vi "DeltaYonDeltaX.vi"() -> (0 "New Values In":string[][](array[string])=[["Test data5"]], 1 "New Chs In":string[](array[string])=["30-10-03:New:Channel new5"])   [LabVIEW 2022 SP3]
uses:
  Results_plotter_Global.vi
  Data plotting/subVIs/Plot_Values_Global.vi
panel:
  # "Similar to Calculate_Gradient.vi, but also returns sign. However does not cope with multiple ordinates."
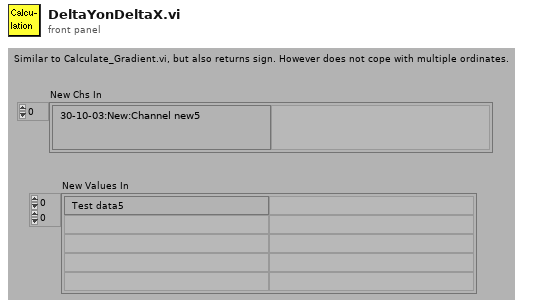
[diagram p1: front panel]
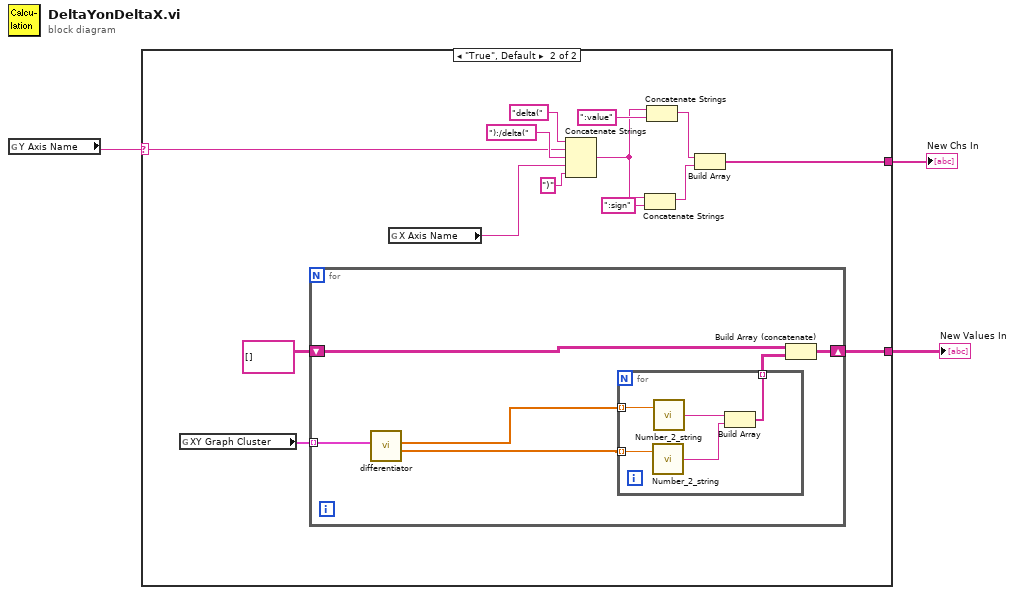
[diagram p0: block diagram]
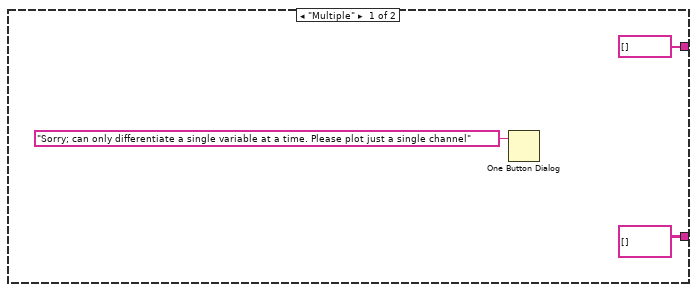
[diagram p2: hidden frame]
diagram:
  n1 = global read "Results_plotter_Global.vi" "Y Axis Name"() -> (w1:string)
  n2 = case shown="\"True\", Default" w1 {
    selector: w1 -> [_ w7]
    tunnel: [string[][] [] w19] -> w3
    tunnel: [string[] [] w11] -> w2
    frame "Multiple" {
      n3 = One Button Dialog(message="Sorry; can only differentiate a single variable at a time. Please plot just a single channel") -> ()  [unwired: 1 in, 1 out]
    }
    frame "True", Default {
      n4 = global read "Plot_Values_Global.vi" "XY Graph Cluster"() -> (w18:cluster{dbl[], dbl[]}[])
      n5 = for {
        tunnel: w18 -> [w23] mode=indexing
        shift-right: [w24] -> w19
        shift-left: string[][] [] -> [w26]
        n6 = call "differentiator.vi"("X-YCluster"=w23) -> ("sign"=w21:dbl[], "deltaY/deltaX"=w22:dbl[])  [unwired: 9 in]
        n7 = for {
          tunnel: w21 -> [w29] mode=indexing
          tunnel: [w30] -> w25 mode=indexing
          tunnel: w22 -> [w28] mode=indexing
          n8 = call "Number_2_string.vi"("number"=w29) -> ("String"=w31:string)  [unwired: 1 in]
          n9 = call "Number_2_string.vi"("number"=w28) -> ("String"=w27:string)  [unwired: 1 in]
          n10 = Build Array(w27, w31) -> (w30:string[])
        }
        n11 = Build Array (concatenate)(w26, w25) -> (w24:string[][])
      }
      n12 = global read "Results_plotter_Global.vi" "X Axis Name"() -> (w12:string)
      n13 = Concatenate Strings("delta(" ("string"), w7, "):/delta(" ("string"), w12, ")" ("string")) -> (w9:string)
      n14 = Concatenate Strings(w9, ":sign" ("string")) -> (w17:string)
      n15 = Concatenate Strings(w9, ":value" ("string")) -> (w8:string)
      n16 = Build Array(w8, w17) -> (w11:string[])
    }
  }
  "New Chs In" <- w2
  "New Values In" <- w3
